vi "Call Dynamic.vi"(8 "error in":errorcluster, 11 "VI Path":path) -> (0 "error out":errorcluster)   [LabVIEW 2020]
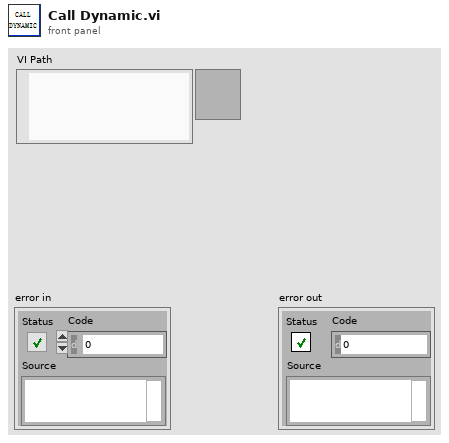
[diagram p1: front panel]
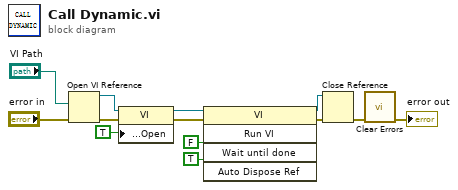
[diagram p0: block diagram]
diagram:
  n1 = Open VI Reference(vi path="VI Path", error in (no error)="error in") -> (vi reference=w13:refnum<vi>, error out=w10:errorcluster)  [unwired: 4 in]
  n2 = property on="Property Node" class="VI"(reference=w13, error in=w10, "Front Panel Window:Open"=TRUE) -> (reference out=w12:refnum<vi>, error out=w11:errorcluster)
  n3 = invoke class="VI" method="Run VI"(reference=w12, error in=w11, "Wait until done"=FALSE ("结束前等待"), "Auto Dispose Ref"=TRUE ("自动销毁引用")) -> (reference out=w8:refnum<vi>, error out=w7:errorcluster)  [unwired: 1 in, 3 out]
  n4 = Close Reference(reference=w8, error in (no error)=w7) -> (error out=w6:errorcluster)
  n5 = call <vilib>:"Clear Errors.vi"("error in (no error)"=w6) -> ("error out"=→"error out":errorcluster)  [unwired: 5 in, 1 out]
